vi "read_ini.vi"(8 "error in (no error)":errorcluster caption="错误输入（无错误）", 9 "section name":string, 10 "file ref in":T1, 11 "LimitSwitch 输入":refnum<class "LimitSwitch.lvclass">) -> (0 "error out":errorcluster caption="错误输出", 2 "file ref out":T1, 3 "LimitSwitch 输出":refnum<class "LimitSwitch.lvclass">)   [LabVIEW 2016, in "MotionControl.lvlib" / "LimitSwitch.lvclass"]
uses:
  <userlib>/MotionControl/LimitSwitch/LimitSwitch.lvclass
  <vilib>/Utility/config.llb/Config Data RefNum.ctl
  <userlib>/MotionControl/LimitSwitch/LimitSwitch.lvclass/LimitSwitch.ctl
  <vilib>/Utility/config.llb/Read Key (U32).vi
  <vilib>/Utility/config.llb/Read Key (I32).vi
  <vilib>/ErrorRing/Error Ring.xnode
  <vilib>/Utility/config.llb/NI_LVConfig.lvlib
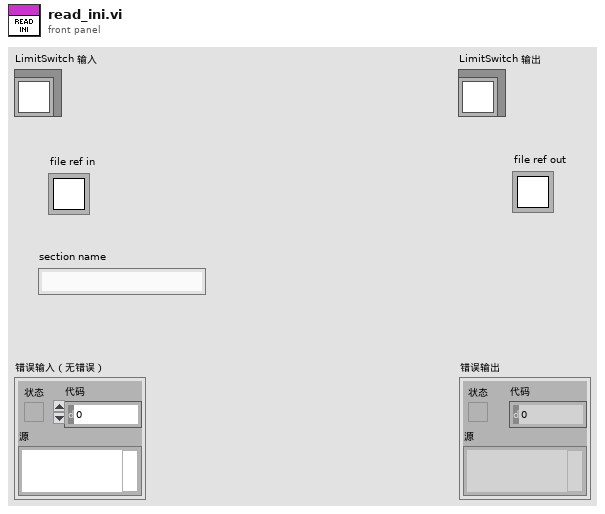
[diagram p1: front panel]
types:
  T1 = typedef "NI_LVConfig.lvlib/Config Data RefNum.ctl" = refnum<k1>
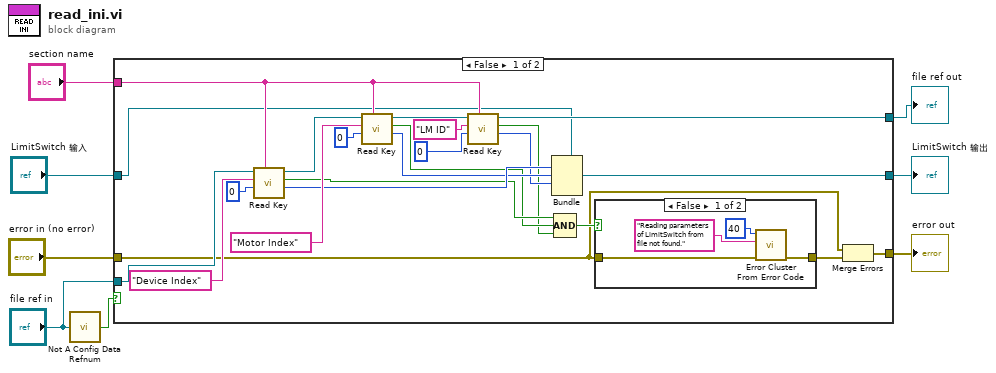
[diagram p0: block diagram]
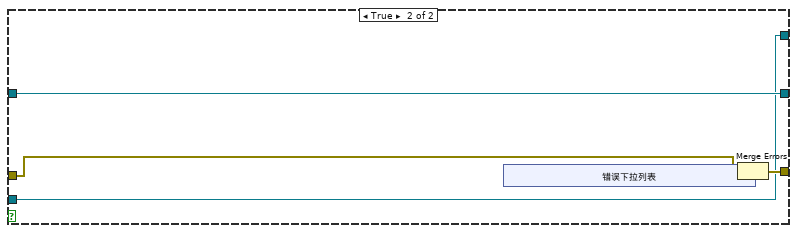
[diagram p3: hidden frame]
diagram:
  n1 = call <vilib>:"Not A Config Data Refnum.vi"("refnum"="file ref in") -> ("not a config data refnum"=w5:bool)
  n2 = case shown="False" w5 {
    tunnel: [w9 w38] -> w8
    tunnel: [w16 w41] -> w6
    tunnel: "LimitSwitch 输入" -> [w17 w41]
    tunnel: "error in (no error)" -> [w11 w39]
    tunnel: "file ref in" -> [w31 w37]
    tunnel: "section name" -> [w27 _]
    tunnel: [w24 w37] -> w1
    frame False {
      n3 = call-poly <vilib>:"Read Key.vi"("section"=w27, "default value"=u32 0, "key"="Device Index", "refnum"=w31) -> ("value"=w20:u32, "found?"=w15:bool, "refnum out"=w29:T1)  [unwired: 4 in, 1 out]
      n4 = call-poly <vilib>:"Read Key.vi"("section"=w27, "default value"=u32 0, "key"="Motor Index", "refnum"=w29) -> ("value"=w19:u32, "found?"=w14:bool, "refnum out"=w28:T1)  [unwired: 4 in, 1 out]
      n5 = call-poly <vilib>:"Read Key.vi"("section"=w27, "default value"=0, "key"="LM ID", "refnum"=w28) -> ("value"=w18:i32, "found?"=w13:bool, "refnum out"=w24:T1)  [unwired: 4 in, 1 out]
      n6 = Bundle(cluster=w17, w20, w19, w18) -> (w16:refnum<class "LimitSwitch.lvclass">)  [unwired: 2 in]
      n7 = Compound Arithmetic op=AND(w15, w14, w13) -> (w12:bool)
      n8 = case shown="False" w12 {
        tunnel: w11 -> [w33 w36]
        tunnel: [w32 w36] -> w10
        frame False {
          n9 = call <vilib>:"Error Cluster From Error Code.vi"("error in (no error)"=w33, "error message (\"\")"="Reading parameters of LimitSwitch from file not found." ("error message (\"\")"), "error code (0)"=40) -> ("error out"=w32:errorcluster)  [unwired: 6 in]
        }
        frame True {
        }
      }
      n10 = Merge Errors(w11, w10) -> (w9:errorcluster)
    }
    frame True {
      n11 = xnode "错误下拉列表"() -> ("error out"=w40:errorcluster)
      n12 = Merge Errors(w39, w40) -> (w38:errorcluster)
    }
  }
  "error out" <- w8
  "LimitSwitch 输出" <- w6
  "file ref out" <- w1
